vi "Create Command Description.vi"(8 "error in (no error)":errorcluster, 11 "Help in":refnum<class "Help.lvclass">) -> (0 "error out":errorcluster, 2 "<JSON> out":string, 3 "Help out":refnum<class "Help.lvclass">)   [LabVIEW 2019, in "Instrument.lvlib" / "Help.lvclass"]
uses:
  Help.lvclass
  Help.lvclass/Help.ctl
  76c6f626-863b-4e4b-88bc-9b29d27459f4.vi
  664a37cf-32ce-49df-980f-cb91fa91d3c6.vi
  <vilib>/JDP Science/JSONtext/Variant to JSON Text.vi
  <vilib>/JDP Science/JSONtext/Set Item.vi
  <vilib>/JDP Science/JSONtext/LVClass Serializer/JSONtext LVClass Serializer.lvclass
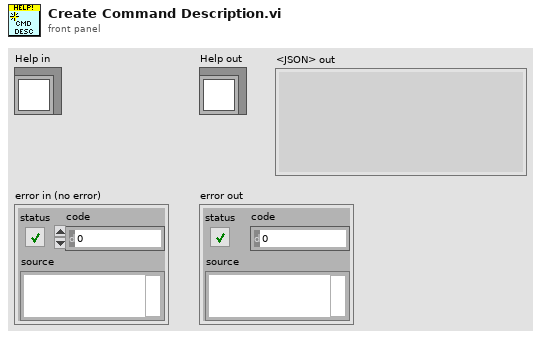
[diagram p1: front panel]
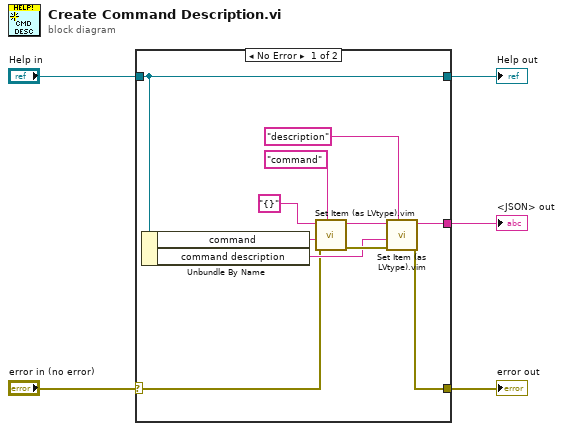
[diagram p0: block diagram]
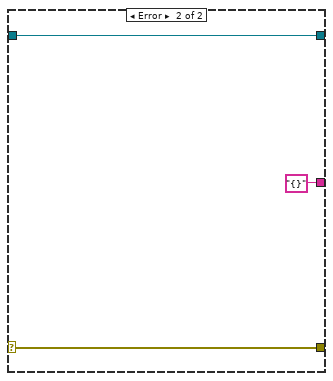
[diagram p2: hidden frame]
diagram:
  n1 = case shown="No Error" "error in (no error)" {
    selector: "error in (no error)" -> [w9 w18]
    tunnel: [w16 "{}" ("JSON")] -> w1
    tunnel: [w15 w18] -> w2
    tunnel: "Help in" -> [w6 w19]
    tunnel: [w6 w19] -> w5
    frame No Error {
      n2 = Unbundle By Name(w6) -> ("command"=w8:string, "command description"=w10:string)
      n3 = call "Set Item (as LVtype).vim"("$Path or Item Name"="command", "error in (no error)"=w9, "Anything"=w8, "JSON"="{}") -> ("error out"=w11:errorcluster, "<JSON>"=w14:string)  [unwired: 4 in, 1 out]
      n4 = call "Set Item (as LVtype).vim"("$Path or Item Name"="description", "error in (no error)"=w11, "Anything"=w10, "JSON"=w14) -> ("error out"=w15:errorcluster, "<JSON>"=w16:string)  [unwired: 4 in, 1 out]
    }
    frame Error {
    }
  }
  "Help out" <- w5
  "error out" <- w2
  "<JSON> out" <- w1
